vi "Keep Printable Characters.vi"(1 "String in":string) -> (0 "String out (printable characters only - ASCII 0x20 to 0x7F)":string)   [LabVIEW 2020, in "Error Manager.lvlib"]
doc: "Traverses the input string and filters (keeps) all Printable Characters. The output string is like the input string, but with some characters removed.\n\nASCII table: http://www.asciitable.com/\n\nPerformance: This VI is inlined to increase performance"
uses:
  Error Manager.lvlib
panel:
  # "Development\ncontrols/indicators useful for development and testing, but which are not outputs of the VI"
  # "Input\nInputs to the VI"
  # "Output\nOutputs of the VI"
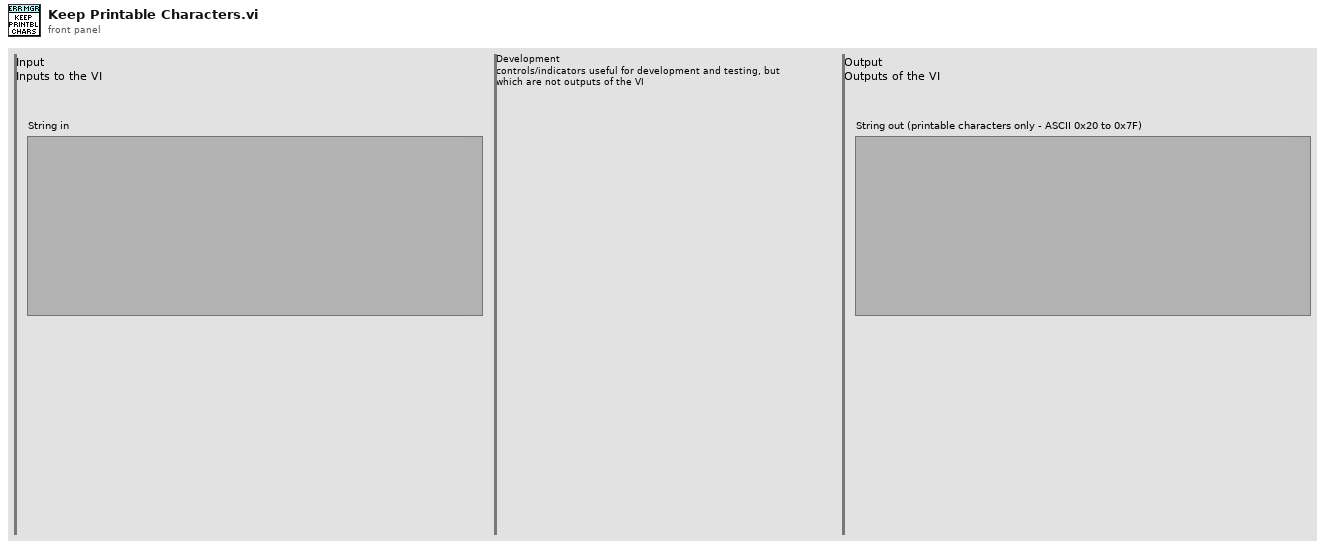
[diagram p1: front panel]
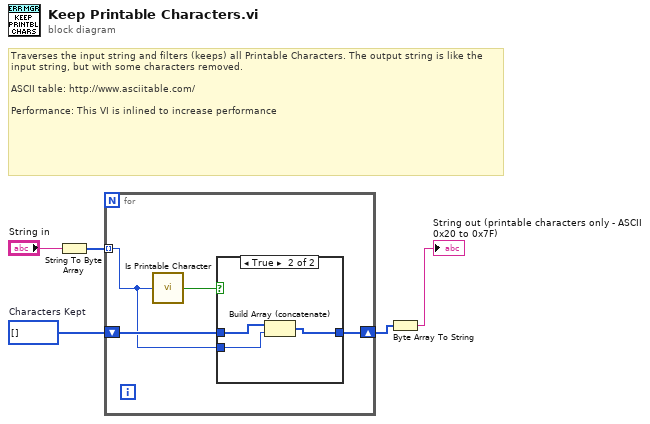
[diagram p0: block diagram]
diagram:
  w3 = u8[] []  # Characters Kept
  # "Traverses the input string and filters (keeps) all Printable Characters. The output string is like the input string, but with some characters removed.\n\nASCII table: http://www.asciitable.com/\n\nPerformance: This VI is inlined to increase performance"
  n1 = String To Byte Array(string="String in") -> (unsigned byte array=w4:u8[])
  n2 = for {
    tunnel: w4 -> [w7] mode=indexing
    shift-right: [w6] -> w2
    shift-left: w3 -> [w8]
    n3 = call "Is Printable Character.vi"("ASCII character"=w7) -> ("True = the input is a Printable ASCII character (0x20 to 0x7F)"=w9:bool)
    n4 = case shown="True" w9 {
      tunnel: w8 -> [w10 w13]
      tunnel: w7 -> [_ w12]
      tunnel: [w10 w11] -> w6
      frame False {
      }
      frame True {
        n5 = Build Array (concatenate)(w13, w12) -> (w11:u8[])
      }
    }
  }
  n6 = Byte Array To String(unsigned byte array=w2) -> (string=→"String out (printable characters only - ASCII 0x20 to 0x7F)":string)
